vi "Adjust lvclass ICON.vi"(6 "Debug":bool, 8 "error in":errorcluster, 10 "Overlay Icon":refnum<class "Icon.lvclass">, 11 "Name to Lib Map":map{string, refnum<vi>}(c390)) -> (0 "error out":errorcluster caption="error in", 3 "Name to Lib Map out":map{string, refnum<vi>}(c390), 4 "Result for debugging":cluster{"Name":string, picture[]}[](array[cluster]))   [LabVIEW 2023, in "Plugin Generator.lvlib"]
uses:
  Plugin Generator.lvlib
  <vilib>/LabVIEW Icon API/lv_icon/Classes/Icon/Icon.lvclass
  <vilib>/LabVIEW Icon API/Support/Get Data from Icon Class.vi
  <vilib>/LabVIEW Icon API/lv_icon/Classes/Layer/Substitute Layer.vi
  <vilib>/LabVIEW Icon API/Support/Get Icon Class from Data.vi
  <vilib>/LabVIEW Icon API/Set VI Icon.vi
  <vilib>/LabVIEW Icon API/LabVIEW Icon API.lvlib
  <vilib>/LabVIEW Icon API/Set Text Icon/Text-Based VI Icon.lvlib
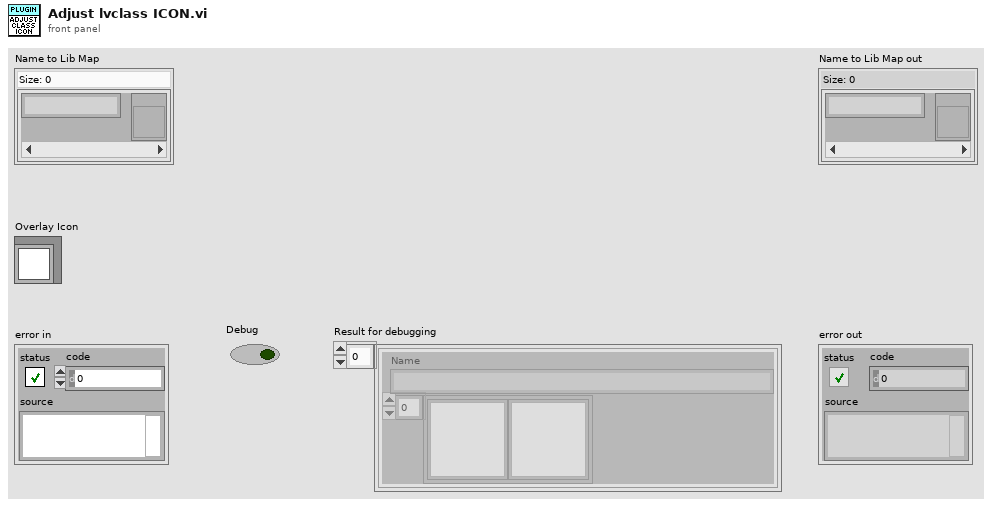
[diagram p1: front panel]
types:
  T1 = typedef "imagedata.ctl" = cluster{"image type":i32, "image depth":i32, "image":u8[], "mask":u8[], "colors":u32[], "Rectangle":cluster{"left":i16, "top":i16, "right":i16, "bottom":i16}}
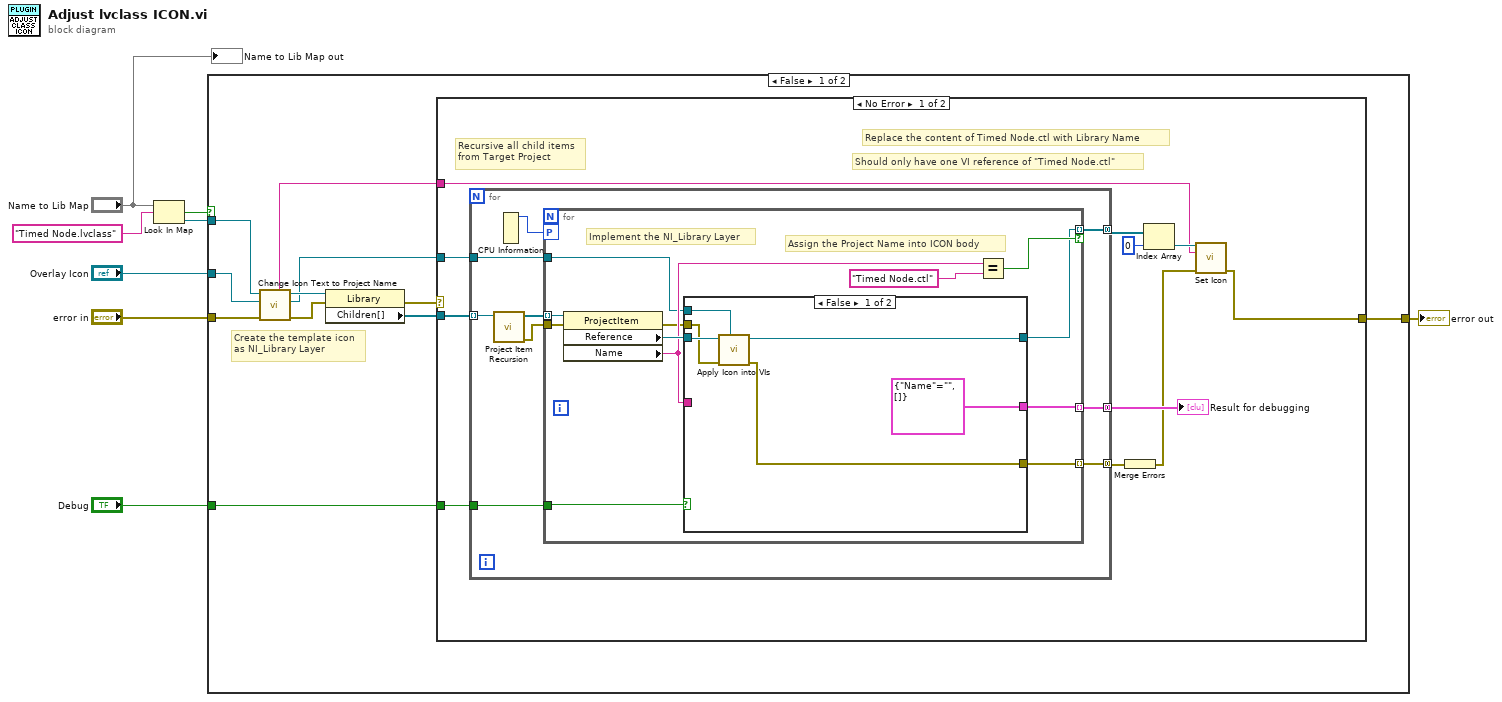
[diagram p0: block diagram]
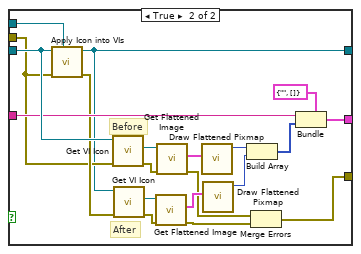
[diagram p2: hidden frame]
diagram:
  n1 = Look In Map(map="Name to Lib Map", key="Timed Node.lvclass" ("String")) -> (key not found?=w6:bool, value=w5:refnum<vi>)  [unwired: 1 in]
  n2 = case shown="False" w6 {
    tunnel: w5 -> [w18 _]
    tunnel: "Debug" -> [w15 _]
    tunnel: "error in" -> [w14 w79]
    tunnel: [w13 w79] -> w2
    tunnel: "Overlay Icon" -> [w10 _]
    frame False {
      # "Create the template icon\nas NI_Library Layer"
      n3 = call "Change Icon Text to Project Name.vi"("error in"=w14, "Overlay Icon"=w10, "Lvclass Ref in"=w18) -> ("error out"=w17:errorcluster, "Layer.lvclass out"=w11:refnum<class "Layer.lvclass">, "Lvclass Ref out"=w12:refnum<vi>, "Body Text.Line 1 text"=w9:string)  [unwired: 5 in]
      n4 = property class="Library"(reference=w12, error in=w17) -> (error out=w16:errorcluster, "Children[]"=w19:refnum<vi>[])  [unwired: 1 out]
      n5 = case shown="No Error" w16 {
        selector: w16 -> [_ w78]
        tunnel: w19 -> [w30 _]
        tunnel: w11 -> [w28 _]
        tunnel: w15 -> [w27 _]
        tunnel: [w21 w78] -> w13
        tunnel: w9 -> [w20 _]
        frame No Error {
          # "Replace the content of Timed Node.ctl with Library Name"
          # "Recursive all child items\nfrom Target Project"
          # "Should only have one VI reference of \"Timed Node.ctl\""
          n6 = for {
            tunnel: w30 -> [w39] mode=indexing
            tunnel: [w37] -> w29 mode=concatenating
            tunnel: w28 -> [w35]
            tunnel: w27 -> [w33]
            tunnel: [w32] -> w26 mode=concatenating
            tunnel: [w31] -> w23 mode=concatenating
            n7 = call "Project Item Recursion.vi"("TargetItem in"=w39) -> ("error out"=w36:errorcluster, "TargetItem out"=w38:refnum<vi>[])  [unwired: 9 in]
            n8 = CPU Information() -> (4:w34:i32)  [unwired: 3 out]
            n9 = for {
              tunnel: w38 -> [w51] mode=indexing
              tunnel: w36 -> [w50]
              tunnel: [w49] -> w37 mode=indexing
              tunnel: w35 -> [w41]
              workers-P: w34 -> [_]
              tunnel: w33 -> [w42]
              tunnel: [w40] -> w32 mode=indexing if=w45
              tunnel: [w44] -> w31 mode=indexing
              # "Implement the NI_Library Layer"
              # "Assign the Project Name into ICON body"
              n10 = property class="ProjectItem"(reference=w51, error in=w50) -> (error out=w43:errorcluster, "Reference"=w48:refnum<vi>, "Name"=w47:string)  [unwired: 1 out]
              n11 = case shown="False" w42 {
                tunnel: [cluster{"Name":string, picture[]} {"Name"="", []} ("cluster") w77] -> w49
                tunnel: w48 -> [w57 w76]
                tunnel: w47 -> [_ w75]
                tunnel: [w54 w73] -> w44
                tunnel: w43 -> [w56 w60]
                tunnel: w41 -> [w55 w59]
                tunnel: [w52 w58] -> w40
                frame False {
                  n12 = call "Apply Icon into VIs.vi"("Substitute Layer"=w55, "error in"=w56, "VI in"=w57) -> ("error out"=w54:errorcluster, "VI Refnum out"=w52:refnum<vi>)  [unwired: 7 in]
                }
                frame True {
                  # "After"
                  # "Before"
                  n13 = call "Apply Icon into VIs.vi"("Substitute Layer"=w59, "error in"=w60, "VI in"=w76) -> ("error out"=w74:errorcluster, "VI Refnum out"=w58:refnum<vi>)  [unwired: 7 in]
                  n14 = call <vilib>:"Get VI Icon.vi"("error in (no error)"=w60, "VI Refnum in"=w76) -> ("error out"=w64:errorcluster, "Icon"=w70:refnum<class "Icon.lvclass">)  [unwired: 7 in, 1 out]
                  n15 = call <vilib>:"Get VI Icon.vi"("error in (no error)"=w74, "VI Refnum in"=w58) -> ("error out"=w63:errorcluster, "Icon"=w72:refnum<class "Icon.lvclass">)  [unwired: 7 in, 1 out]
                  n16 = call <vilib>:"Get Flattened Image.vi"("error in (no error)"=w63, "lv_icon.lvlib:Icon.lvclass in"=w72) -> ("error out"=w61:errorcluster, "Color Image"=w71:T1)  [unwired: 6 in, 2 out]
                  n17 = call <vilib>:"Get Flattened Image.vi"("error in (no error)"=w64, "lv_icon.lvlib:Icon.lvclass in"=w70) -> ("error out"=w62:errorcluster, "Color Image"=w69:T1)  [unwired: 6 in, 2 out]
                  n18 = call <vilib>:"Draw Flattened Pixmap.vi"("image data"=w69) -> ("new picture"=w68:picture)  [unwired: 8 in]
                  n19 = call <vilib>:"Draw Flattened Pixmap.vi"("image data"=w71) -> ("new picture"=w67:picture)  [unwired: 8 in]
                  n20 = Build Array(w68, w67) -> (w66:picture[])
                  n21 = Merge Errors(w62, w61) -> (w73:errorcluster)
                  n22 = Bundle(cluster=cluster{"Name":string, picture[]} {"Name"="", []}, "Name"=w75, w66) -> (w77:cluster{"Name":string, picture[]})
                }
              }
              n23 = Equal?(x=w47, y="Timed Node.ctl" ("x")) -> (x = y?=w45:bool)
            }
          }
          "Result for debugging" <- w29
          n24 = Merge Errors(w23) -> (w22:errorcluster)
          n25 = Index Array(array=w26, index=0) -> (element=w24:refnum<vi>)
          n26 = call <vilib>:"Set Icon.vi"("VI"=w24, "user-supplied text (\"\" - use VI file name)"=w20, "error in"=w22) -> ("error out"=w21:errorcluster)  [unwired: 11 in, 1 out]
        }
        frame Error {
        }
      }
    }
    frame True {
    }
  }
  "error out" <- w2
  "Name to Lib Map out" <- "Name to Lib Map"
